vi "Int32比较选择器（CDB）.vi"(0 "输入1":cdb, 1 "阙值":i32, 2 "信号":i32, 3 "输入2":cdb, 4 "模式":enum16{"≠", "＝", "＞", "≥", "＜", "≤"}(ring)) -> (7 "输出":cdb)   [LabVIEW 2011]
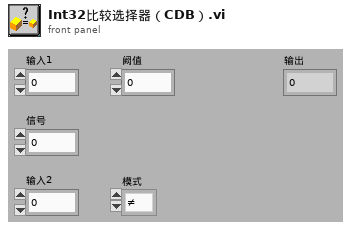
[diagram p1: front panel]
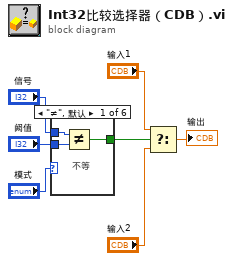
[diagram p0: block diagram]
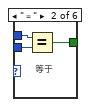
[diagram p2: hidden frame]
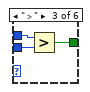
[diagram p3: hidden frame]
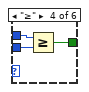
[diagram p4: hidden frame]
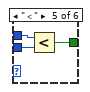
[diagram p5: hidden frame]
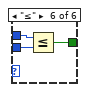
[diagram p6: hidden frame]
diagram:
  n1 = case shown="\"≠\", 默认" "模式" {
    tunnel: "阙值" -> [w9 w11 w16 w19 w22 w25]
    tunnel: "信号" -> [w10 w12 w15 w18 w21 w24]
    tunnel: [w8 w13 w14 w17 w20 w23] -> w5
    frame "≠", Default {
      # "不等"
      n2 = Not Equal?(x=w10, y=w9) -> (x != y?=w8:bool)
    }
    frame "＝" {
      # "等于"
      n3 = Equal?(x=w12, y=w11) -> (x = y?=w13:bool)
    }
    frame "＞" {
      n4 = Greater?(x=w15, y=w16) -> (0:w14:bool)
    }
    frame "≥" {
      n5 = Greater Or Equal?(x=w18, y=w19) -> (x >= y?=w17:bool)
    }
    frame "＜" {
      n6 = Less?(x=w21, y=w22) -> (x < y?=w20:bool)
    }
    frame "≤" {
      n7 = Less Or Equal?(x=w24, y=w25) -> (x <= y?=w23:bool)
    }
  }
  n8 = Select(t="输入1", s=w5, f="输入2") -> (s? t:f=→"输出":cdb)
